vi "PH_AWG-510.PSDB Output Settings.vi"(0 "i ref in":refnum<vi>, 5 "error IO":errorcluster) -> (14 "i ref out":refnum<vi>, 15 "Output Settings PSDB String Data":T1[](array[typedef]), 16 "Output Settings PSDB Numeric Data":T2[](array[typedef]), 17 "Output Settings PSDB 2D Data":T3[](array[typedef]), 18 "Output Settings PSDB Boolean Data":T5[](array[typedef]), 19 "error out":errorcluster)   [LabVIEW 2014, in "PH_AWG-510.lvlib"]
doc: "This VI sets the data of the output settings for the PSDB."
uses:
  PH_AWG-510.lvlib
  PH_Basics/PH_PSDBWriter/PH_PSDBWriter.Boolean dataset.ctl
  PH_Basics/PH_PSDBWriter/PH_PSDBWriter.2D dataset.ctl
  CSlibraries-extern/psdb_lv/PSDB_AxisDescription.ctl
  PH_Basics/PH_PSDBWriter/PH_PSDBWriter.Numeric dataset.ctl
  PH_Basics/PH_PSDBWriter/PH_PSDBWriter.String dataset.ctl
  CSlibraries-extern/psdb_lv/PSDB.lvlib
  PH_Basics/PH_PSDBWriter/PH_PSDBWriter.lvlib
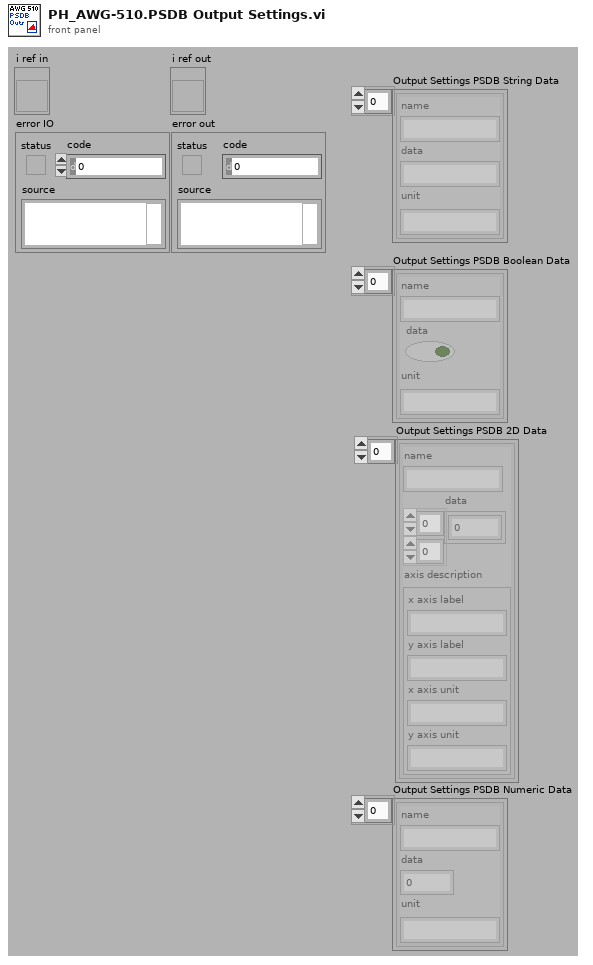
[diagram p1: front panel]
types:
  T1 = typedef "PH_PSDBWriter.lvlib/PH_PSDBWriter.String dataset.ctl" = cluster{"name":string, "data":string, "unit":string}
  T2 = typedef "PH_PSDBWriter.lvlib/PH_PSDBWriter.Numeric dataset.ctl" = cluster{"name":string, "data":dbl, "unit":string}
  T3 = typedef "PH_PSDBWriter.lvlib/PH_PSDBWriter.2D dataset.ctl" = cluster{"name":string, "data":dbl[][], "axis description":T4}
  T4 = typedef "PSDB.lvlib/PSDB_AxisDescription.ctl" = cluster{"x axis label":string, "y axis label":string, "x axis unit":string, "y axis unit":string}
  T5 = typedef "PH_PSDBWriter.lvlib/PH_PSDBWriter.Boolean dataset.ctl" = cluster{"name":string, "data":bool, "unit":string}
  T6 = typedef "PH_AWG-510.lvlib/PH_AWG-510.i attribute.ctl" = cluster{"GUI Refs":cluster{"Delete":refnum<vi>, "Trigger Settings":refnum<vi>, "Start Device":refnum<vi>, "Instrument Information":refnum<vi>, "Lock Frontpanel":refnum<vi>, "Waveform Pattern File":refnum<vi>, "Initialize":refnum<vi>, "Output Settings":refnum<vi>}, "Instrument Information":T7, "Initialized?":bool, "Current Settings":cluster{"Trigger":T8, "Output Settings":T9}, "Wanted Settings":cluster{"Trigger":T8, "Output Settings":T9}, "Device frontpanel locked?":bool, "Default File Path":path}
  T7 = typedef "PH_AWG-510.lvlib/PH_AWG-510.Instrument Information Dataset.ctl" = cluster{"VISA resource name":refnum<visa-resource-name>, "Instrument Firmware Revision":string, "Manufacturer":string, "Model":string, "Serial Number":string, "Error Message":string, "Device Status":enum16{"stopped", "wating for trigger", "running", "Failure"}}
  T8 = typedef "PH_AWG-510.lvlib/PH_AWG-510.Trigger Settings.ctl" = cluster{"Mode":enum16{"Continuous", "Triggered", "Gated", "Enhanced"}, "Level (V)":dbl, "External Source":bool}
  T9 = typedef "PH_AWG-510.lvlib/PH_AWG-510.Output Settings.ctl" = cluster{"Activate Channel":bool, "VPP (V)":dbl, "Clock (Hz)":dbl, "File Name (Device)":string, "#1":u16, "#2":u16, "#3":u16, "#4":u16, "#5":u16, "#6":u16, "#7":u16, "#8":u16, "#9":u16, "#10":u16, "#11":u16, "#12":u16, "#13":u16, "#14":u16, "#15":u16, "#16":u16, "#17":u16, "#18":u16, "#19":u16, "#20":u16, "Offset (V)":dbl}
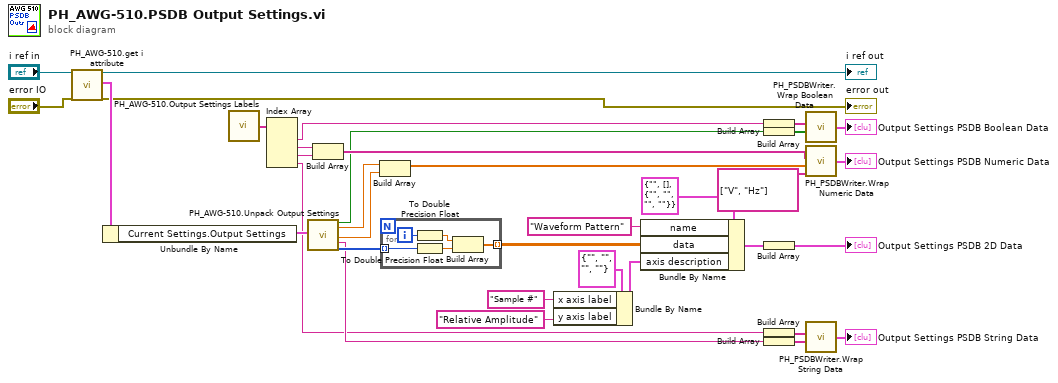
[diagram p0: block diagram]
diagram:
  n1 = call "PH_AWG-510.get i attribute.vi"("i ref in"="i ref in", "error in (no error)"="error IO") -> ("i ref out"=→"i ref out":refnum<vi>, "i attribute"=w33:T6, "error out"=→"error out":errorcluster)  [unwired: 15 in]
  n2 = Unbundle By Name(w33) -> ("Current Settings.Output Settings"=w19:T9)
  n3 = call "PH_AWG-510.Output Settings Labels.vi"() -> ("Output Settings Labels"=w16:string[])
  n4 = Index Array(array=w16) -> (element #1=w11:string, element #2=w15:string, element #3=w14:string, element #4=w1:string)  [unwired: 4 in]
  n5 = call "PH_AWG-510.Unpack Output Settings.vi"("Output Settings"=w19) -> ("Activate Channel"=w7:bool, "VPP [V]"=w6:dbl, "Clock [Hz]"=w5:dbl, "File Name (Device)"=w4:string, "Waveform Pattern"=w18:u16[])  [unwired: 14 in]
  n6 = Build Array(w15, w14) -> (w8:string[])
  n7 = Build Array(w6, w5) -> (w25:dbl[])
  n8 = for {
    tunnel: w18 -> [w40] mode=indexing
    tunnel: [w38] -> w27 mode=indexing
    i -> [w39]
    n9 = To Double Precision Float(number=w39) -> (double precision float=w36:dbl)
    n10 = To Double Precision Float(number=w40) -> (double precision float=w37:dbl)
    n11 = Build Array(w36, w37) -> (w38:dbl[])
  }
  n12 = Bundle By Name(cluster=T4 {"x axis label"="", "y axis label"="", "x axis unit"="", "y axis unit"=""} ("axis description"), "x axis label"="Sample #", "y axis label"="Relative Amplitude") -> (w22:T4)
  n13 = Bundle By Name(cluster=T3 {"name"="", "data"=[], "axis description"={"x axis label"="", "y axis label"="", "x axis unit"="", "y axis unit"=""}} ("2D data"), "name"="Waveform Pattern", "data"=w27, "axis description"=w22) -> (w29:T3)
  n14 = Build Array(w11) -> (w13:string[])
  n15 = Build Array(w7) -> (w17:bool[])
  n16 = Build Array(w29) -> (→"Output Settings PSDB 2D Data":T3[])
  n17 = Build Array(w1) -> (w12:string[])
  n18 = Build Array(w4) -> (w32:string[])
  n19 = call "PH_PSDBWriter.Wrap Boolean Data.vi"("Data Array"=w17, "Name Array"=w13) -> ("PSDB Boolean Data Array"=→"Output Settings PSDB Boolean Data":T5[])  [unwired: 2 in]
  n20 = call "PH_PSDBWriter.Wrap Numeric Data.vi"("Unit Array"=string[] ["V", "Hz"], "Data Array"=w25, "Name Array"=w8) -> ("PSDB Numeric Data Array"=→"Output Settings PSDB Numeric Data":T2[])  [unwired: 1 in]
  n21 = call "PH_PSDBWriter.Wrap String Data.vi"("Data Array"=w32, "Name Array"=w12) -> ("PSDB String Data Array"=→"Output Settings PSDB String Data":T1[])  [unwired: 2 in]
